vi "Acquire3.vi"() -> ()   [LabVIEW 2022 SP3]
uses:
  <vilib>/DAQmx/read.llb/DAQmx Read (Analog Wfm 1Chan NSamp).vi
  <vilib>/Analysis/baseanly.llb/Mean (DBL).vi
  <vilib>/DAQmx/write.llb/DAQmx Write (Digital 1D Bool NChan 1Samp 1Line).vi
  Global 1.vi
  <vilib>/DAQmx/create/channels.llb/DAQmx Create Channel (DO-Digital Output).vi
  <vilib>/DAQmx/create/channels.llb/DAQmx Create Channel (AI-Voltage-Basic).vi
  <vilib>/DAQmx/configure/timing.llb/DAQmx Timing (Sample Clock).vi
  <vilib>/DAQmx/miscellaneous.llb/DAQmx Fill In Error Info.vi
  <vilib>/Analysis/NI_AALBase.lvlib
panel:
  out "Numeric 3":dbl
  out "Numeric 2":dbl
  out "String":string
  out "Numeric":dbl
  in  "stop":bool
  out "Waveform Graph":waveform(dbl)(graph)
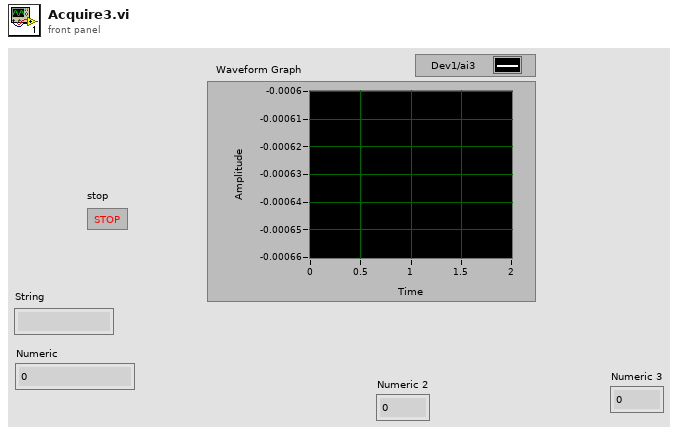
[diagram p1: front panel]
types:
  T1 = typedef "test.ctl" = bool[][]
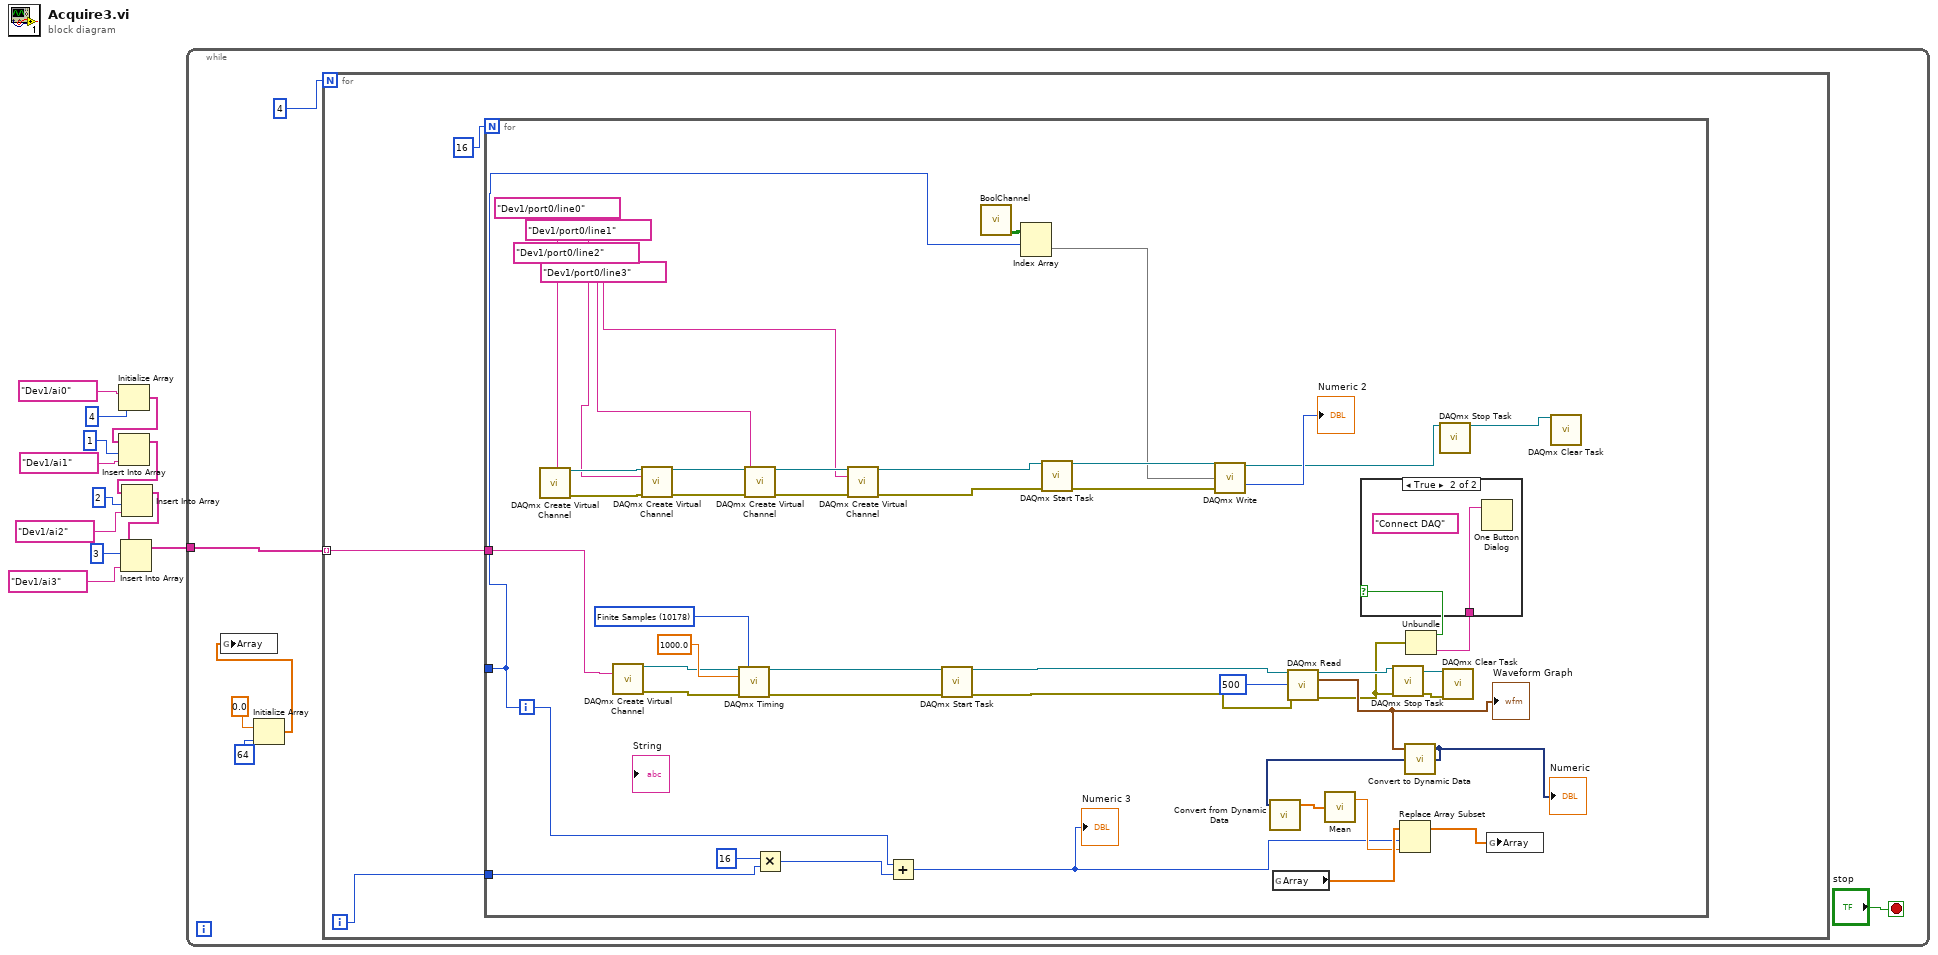
[diagram p0: block diagram]
diagram:
  n1 = Initialize Array(tag "Dev1/ai0" ("physical channels"), 4) -> (w9:tag[])
  n2 = Insert Into Array(array=w9, index=1, new element=tag "Dev1/ai1" ("physical channels")) -> (w7:tag[])
  n3 = Insert Into Array(array=w7, index=2, new element=tag "Dev1/ai2" ("physical channels")) -> (w3:tag[])
  n4 = Insert Into Array(array=w3, index=3, new element=tag "Dev1/ai3" ("physical channels")) -> (w1:tag[])
  n5 = while {
    tunnel: w1 -> [w14]
    stop <- "stop" stop-if-true
    n6 = Initialize Array(0.0, 64) -> (w15:dbl[])
    n7 = global write "Global 1.vi" "Array"(w15) -> ()
    n8 = for {
      N: 4 -> [_]
      tunnel: w14 -> [w20] mode=indexing
      i -> [w19]
      n9 = for {
        N: 16 -> [_]
        tunnel: [w27] -> _
        tunnel: w20 -> [w30]
        tunnel: w19 -> [w25]
        i -> [w27]
        w64 = 10178 items=["Finite Samples"=10178, "Continuous Samples"=10123, "Hardware Timed Single Point"=12522] ("sample mode")
        n10 = call-poly <vilib>:"DAQmx Create Virtual Channel.vi"("lines"=tag "Dev1/port0/line0") -> ("task out"=w43:refnum<k21>, "error out"=w41:errorcluster)  [unwired: 13 in]
        n11 = call-poly <vilib>:"DAQmx Create Virtual Channel.vi"("physical channels"=w30) -> ("task out"=w28:refnum<k21>, "error out"=w29:errorcluster)  [unwired: 13 in]
        n12 = call-poly <vilib>:"DAQmx Create Virtual Channel.vi"("task in"=w43, "lines"=tag "Dev1/port0/line1", "error in"=w41) -> ("task out"=w38:refnum<k21>, "error out"=w40:errorcluster)  [unwired: 11 in]
        n13 = call-poly <vilib>:"DAQmx Timing.vi"("task/channels in"=w28, "sample mode"=w64, "rate"=1000.0, "error in"=w29) -> ("task out"=w57:refnum<k21>, "error out"=w56:errorcluster)  [unwired: 10 in]
        n14 = call-poly <vilib>:"DAQmx Create Virtual Channel.vi"("task in"=w38, "lines"=tag "Dev1/port0/line2", "error in"=w40) -> ("task out"=w37:refnum<k21>, "error out"=w39:errorcluster)  [unwired: 11 in]
        n15 = Multiply(x=16, y=w25) -> (x*y=w24:i32)
        n16 = call-poly <vilib>:"DAQmx Create Virtual Channel.vi"("task in"=w37, "lines"=tag "Dev1/port0/line3", "error in"=w39) -> ("task out"=w36:refnum<k21>, "error out"=w35:errorcluster)  [unwired: 11 in]
        n17 = Add(x=w27, y=w24) -> (x+y=w23:i32)
        "Numeric 3" <- w23
        n18 = call <vilib>:"DAQmx Start Task.vi"("task/channels in"=w57, "error in"=w56) -> ("task out"=w55:refnum<k21>, "error out"=w54:errorcluster)  [unwired: 12 in]
        n19 = call "BoolChannel.vi"() -> ("Array"=w32:T1)  [unwired: 11 in]
        n20 = Index Array(array=w32, index (row)=w27) -> (element=w31:bool[])  [unwired: 1 in]
        n21 = call <vilib>:"DAQmx Start Task.vi"("task/channels in"=w36, "error in"=w35) -> ("task out"=w46:refnum<k21>, "error out"=w52:errorcluster)  [unwired: 12 in]
        n22 = call-poly <vilib>:"DAQmx Write.vi"("task/channels in"=w46, "data"=w31, "error in"=w52) -> ("task out"=w44:refnum<k21>, "number of samples written per channel"=→"Numeric 2":u32)  [unwired: 10 in, 1 out]
        n23 = global read "Global 1.vi" "Array"() -> (w60:dbl[])
        n24 = call-poly <vilib>:"DAQmx Read.vi"("task/channels in"=w55, "number of samples per channel"=500, "error in"=w54) -> ("task out"=w48:refnum<k21>, "data"=w63:waveform(dbl), "error out"=w47:errorcluster)  [unwired: 10 in]
        "Waveform Graph" <- w63
        n25 = call <vilib>:"DAQmx Stop Task.vi"("task/channels in"=w48, "error in"=w47) -> ("task out"=w49:refnum<k21>, "error out"=w50:errorcluster)  [unwired: 12 in]
        n26 = call "Convert to Dynamic Data"("Waveform"=w63) -> ("Dynamic Data Type"=w62:dynamicdata)  [unwired: 3 in]
        "Numeric" <- w62
        n27 = call "Convert from Dynamic Data"("Dynamic Data Type"=w62) -> ("Array"=w61:dbl[])  [unwired: 3 in]
        n28 = call-poly <vilib>:"Mean.vi"("X"=w61) -> ("mean"=w59:dbl)  [unwired: 1 out]
        n29 = Replace Array Subset(array=w60, new element=w59, index=w23) -> (w22:dbl[])
        n30 = Unbundle(w47) -> ("status"=w66:bool, "source"=w58:string)  [unwired: 1 out]
        n31 = case shown="True" w66 {
          tunnel: w58 -> [_ w68]
          frame False {
          }
          frame True {
            (unwired) "Connect DAQ"
            n32 = One Button Dialog(message=w68) -> ()  [unwired: 1 in, 1 out]
          }
        }
        n33 = call <vilib>:"DAQmx Stop Task.vi"("task/channels in"=w44) -> ("task out"=w45:refnum<k21>)  [unwired: 13 in, 1 out]
        n34 = call <vilib>:"DAQmx Clear Task.vi"("task in"=w49, "error in"=w50) -> ()  [unwired: 13 in, 1 out]
        n35 = global write "Global 1.vi" "Array"(w22) -> ()
        n36 = call <vilib>:"DAQmx Clear Task.vi"("task in"=w45) -> ()  [unwired: 14 in, 1 out]
      }
    }
  }
